vi "Update Plot Name.vi"(8 "error in (no error)":errorcluster, 10 "NewVal":cluster{"String":string, "Picture":picture}[](array[cluster]), 11 "2D Feather.lvclass in":refnum<class "2D Feather.lvclass">) -> (0 "error out":errorcluster, 3 "2D Feather.lvclass out":refnum<class "2D Feather.lvclass">)   [LabVIEW 2017, in "2D Feather.lvclass"]
uses:
  <vilib>/Math Plots/2D Math Plots/2D Feather/2D Feather/2D Feather.lvclass
  <vilib>/Math Plots/2D Math Plots/2D Feather/2D Feather/2D Feather.lvclass/2D Feather.ctl
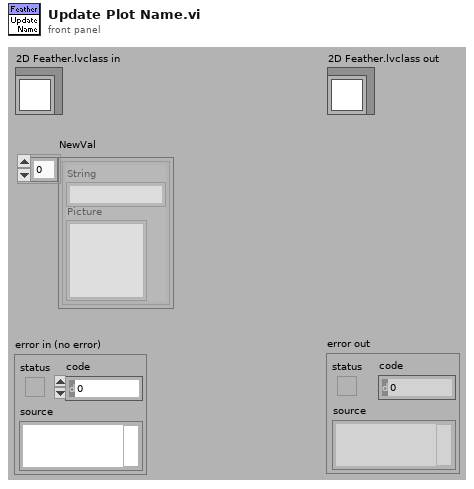
[diagram p1: front panel]
types:
  T1 = typedef "2D Plot.lvclass/Plot Property Array.ctl" = T2[]
  T2 = typedef "2D Plot.lvclass/Plot Property.ctl" = cluster{"Bar Plot Style":u8, "DigitalLineStyle":u8, "TransitionLocation":u8, "Transition Type":u8, "Fill To":i16, "Fill/Pt. Color":u32, "Label Style":u8, "Line Style":u8, "Line Width":u8, "Plot Color":u32, "Plot Interpolation":u8, "Plot Name":string, "Point Style":u8, "Visible?":bool, "XScaleIdx":u32, "YScaleIdx":u32}
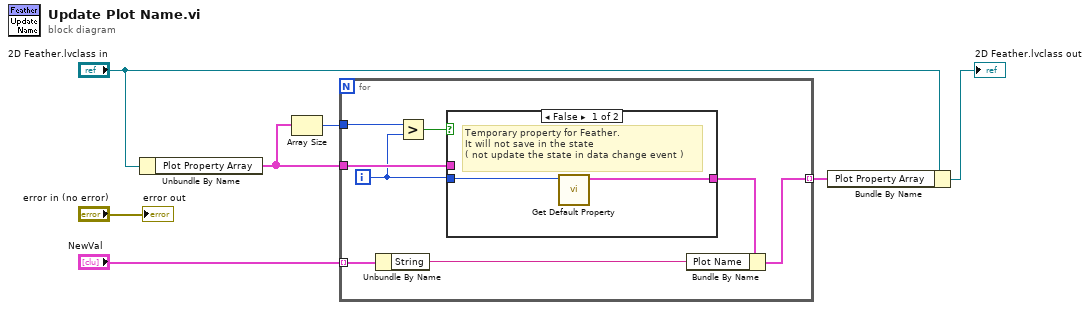
[diagram p0: block diagram]
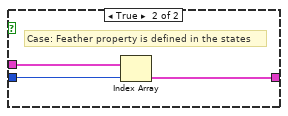
[diagram p2: hidden frame]
diagram:
  n1 = Unbundle By Name("2D Feather.lvclass in") -> ("Plot Property Array"=w6:T1)
  n2 = Array Size(array=w6) -> (size(s)=w7:i32)
  n3 = for {
    tunnel: "NewVal" -> [w14] mode=indexing
    tunnel: w6 -> [w10]
    tunnel: [w15] -> w5 mode=indexing
    tunnel: w7 -> [w11]
    i -> [w8]
    n4 = Unbundle By Name(w14) -> ("String"=w13:string)
    n5 = Greater?(x=w11, y=w8) -> (0:w12:bool)
    n6 = case shown="False" w12 {
      tunnel: w10 -> [_ w20]
      tunnel: w8 -> [w16 w19]
      tunnel: [w17 w18] -> w9
      frame False {
        # "Temporary property for Feather.\nIt will not save in the state\n( not update the state in data change event )"
        n7 = call <vilib>:"Get Default Property.vi"("Index"=w16) -> ("Temporary Property"=w17:T2)  [unwired: 3 in, 7 out]
      }
      frame True {
        # "Case: Feather property is defined in the states"
        n8 = Index Array(array=w20, index=w19) -> (element=w18:T2)
      }
    }
    n9 = Bundle By Name(cluster=w9, "Plot Name"=w13) -> (w15:T2)
  }
  n10 = Bundle By Name(cluster="2D Feather.lvclass in", "Plot Property Array"=w5) -> (→"2D Feather.lvclass out":refnum<class "2D Feather.lvclass">)
  "error out" <- "error in (no error)"
